vi "Main.vi"(11 "Module Admin":refnum<class "Delacor_lib_QMH_Module Admin.lvclass">) -> ()   [LabVIEW 2026, in "Plaintext to CW Sender.lvlib"]
doc: "This template is based off of the Queued Message Handler design pattern and the Queued Message Handler project template that ships with LabVIEW.\n\nThe main difference is that the queue is private to this module and communication between modules is performed via Broadcast and Request events.\n\nRequest events are wrapped in public API methods and are handled in the Event Handling Loop (EHL) of this VI. Any module can register for Broadcast events sent by this module. The EHL generates messages based on user interface actions.\n\nThe Message Handling Loop (MHL) processes messages generated by the EHL, or by other messages. The messages are string values, so new messages can be added easily to the Message Cases case structure in the MHL. Each message cluster can also provide an optional value for Message Data, which is a variant that can be converted to whatever message-specific data is required.\n_____\nBased on DQMH Dev Tools: Project Template 7.1.2.1547."
uses:
  Plaintext to CW Sender.lvlib
  <vilib>/Delacor/Delacor QMH/Libraries/Module Admin_class/Delacor_lib_QMH_Module Admin.lvclass
  Module Data--cluster.ctl
  <vilib>/Dataflow_G/G-Audio/Controls/Audio Device Refnum.ctl
  <vilib>/Delacor/Delacor QMH/Libraries/Message Queue_class/Delacor_lib_QMH_Message Queue.lvclass/Delacor_lib_QMH_Message Queue.ctl
  Stop Argument--cluster.ctl
  <vilib>/Delacor/Delacor QMH/Libraries/Module Admin_class/Delacor_lib_QMH_Module Admin.lvclass/Delacor_lib_QMH_Module Admin.ctl
  Get VI Ref Argument--cluster.ctl
  Get VI Ref (Reply Payload)--cluster.ctl
  <vilib>/Utility/miscctls.llb/LVPointTypeDef.ctl
  <vilib>/Dataflow_G/G-Audio/Controls/Audio Device Info.ctl
  <vilib>/Dataflow_G/G-Audio/Controls/Audio Device Type.ctl
  <vilib>/Dataflow_G/G-Audio/Controls/Audio Device Native Data Format.ctl
  <vilib>/Dataflow_G/G-Audio/Controls/Audio Device Format.ctl
  <vilib>/Dataflow_G/G-Audio/Controls/Audio Device Config.ctl
  <vilib>/Delacor/Delacor QMH/Libraries/Message Queue_class/Delacor_lib_QMH_Enqueue Message (Single).vi
  <vilib>/Delacor/Delacor QMH/Libraries/Module Admin_class/Delacor_lib_QMH_Get External Launch.vi
  28860a4c-ef95-4274-8184-17b162956eb9.vi
  a59a87ba-3734-490d-884d-561db4356e67.vi
  <vilib>/Dataflow_G/G-Audio/Private/Result To Error.vi
  28860a4c-ef95-4274-8184-17b162956eb9.vi/4dfb5711-8d81-45a3-b3db-a84d40650863.vi
  28860a4c-ef95-4274-8184-17b162956eb9.vi/c8869513-30c6-44f2-a2d3-73232fe63870.vi
  <vilib>/Dataflow_G/G-Audio/Private/Audio Device Refnum To Value.vi
  a59a87ba-3734-490d-884d-561db4356e67.vi/4dfb5711-8d81-45a3-b3db-a84d40650863.vi
  a59a87ba-3734-490d-884d-561db4356e67.vi/c8869513-30c6-44f2-a2d3-73232fe63870.vi
  28860a4c-ef95-4274-8184-17b162956eb9.vi/4dfb5711-8d81-45a3-b3db-a84d40650863.vi/4b7b629c-2e91-4160-9820-a26af8f6e677.vi
  28860a4c-ef95-4274-8184-17b162956eb9.vi/c8869513-30c6-44f2-a2d3-73232fe63870.vi/4b7b629c-2e91-4160-9820-a26af8f6e677.vi
  a59a87ba-3734-490d-884d-561db4356e67.vi/4dfb5711-8d81-45a3-b3db-a84d40650863.vi/4b7b629c-2e91-4160-9820-a26af8f6e677.vi
  a59a87ba-3734-490d-884d-561db4356e67.vi/c8869513-30c6-44f2-a2d3-73232fe63870.vi/4b7b629c-2e91-4160-9820-a26af8f6e677.vi
  <vilib>/Utility/Data Type/Get Numeric Information.vi
  <vilib>/Waveform/WDTOps.llb/WDT Waveform Duration DBL.vi
  <vilib>/Delacor/Delacor QMH/Libraries/Message Queue_class/Delacor_lib_QMH_Message Queue.lvclass
  <vilib>/Dataflow_G/G-Audio/G-Audio.lvlib
  FT-818 CW Key Control/FT-818 CW Key Control.lvlib
panel:
  in  "CAT Rate":u32=38400
  in  "Radio Comm Port":refnum<visa-resource-name>
  in  "Connect to FT-818":bool
  out "CW Waveform":waveform(dbl)(graph)
  in  "Unit Speed (sec)":dbl=0.13 min=0.0 max=0.5 step=0.01
  in  "Word Gap":u8=7
  in  "Character Gap":u8=3
  in  "Send":bool
  in  "Preview":bool
  in  "Plaintext":string
  out "error out":errorcluster
  out "Status":string
  in  "Simulate MHL Error":bool
  in  "Simulate EHL Error":bool
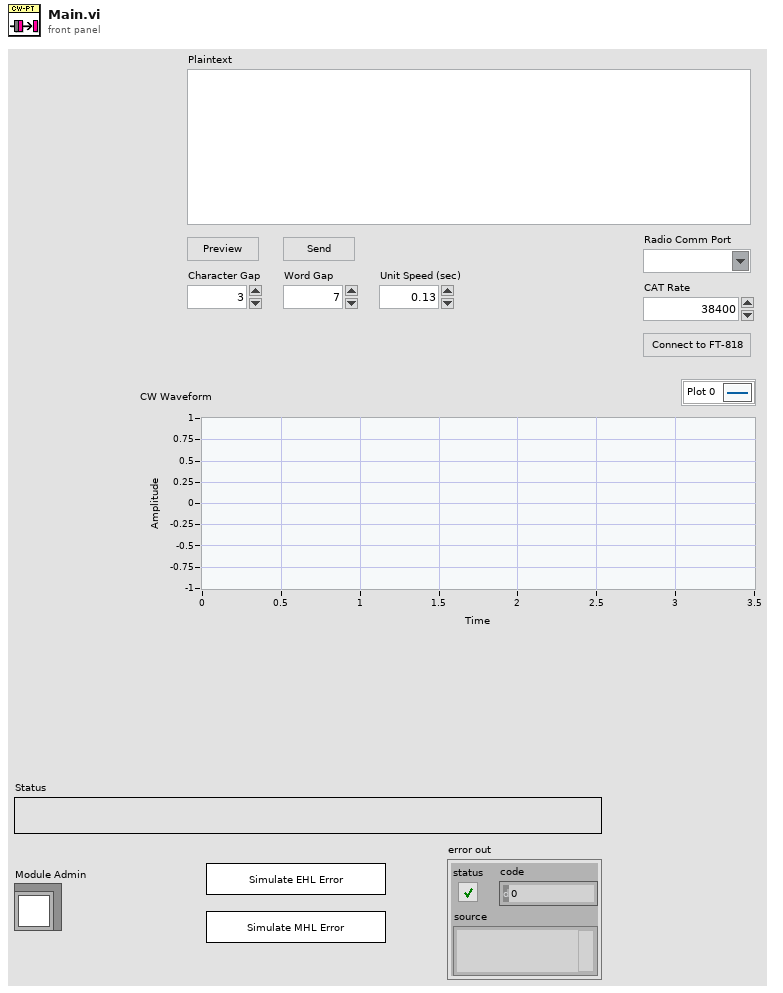
[diagram p1: front panel]
types:
  T1 = typedef "Plaintext to CW Sender.lvlib/Request Events--cluster.ctl" = cluster{"Stop Module":refnum<user-event>, "Show Panel":refnum<user-event>, "Hide Panel":refnum<user-event>, "Get Module Execution Status":refnum<user-event>, "Show Diagram":refnum<user-event>, "Get VI Ref":refnum<user-event>}
  T2 = typedef "FT-818 CW Key Control.lvlib/Broadcast Events--cluster.ctl" = cluster{"Module Did Init":refnum<user-event>, "Status Updated":refnum<user-event>, "Error Reported":refnum<user-event>, "Module Did Stop":refnum<user-event>, "Update Module Execution Status":refnum<user-event>}
  T3 = typedef "Plaintext to CW Sender.lvlib/Module Data--cluster.ctl" = cluster{"Status":string, "Plaintext to CW Map":map{string, bool[]}, "Audio Dev Ref":T4}
  T4 = typedef "G-Audio.lvlib/Audio Device Refnum.ctl" = refnum<file>
  T5 = enum32{"invalid lock state", "Not Locked", "Locked (No Password)", "Password-protected"}
  T6 = typedef "Plaintext to CW Sender.lvlib/Stop Argument--cluster.ctl" = cluster{"Origin":string, "Exit via Stop Module Req?":bool, "Wait for Module to stop?":bool}
  T7 = typedef "Plaintext to CW Sender.lvlib/Get VI Ref Argument--cluster.ctl" = cluster{"Wait Notifier":refnum<notifier>, "wait for reply":bool}
  T8 = typedef "LVPointTypeDef.ctl" = cluster{"Horizontal":i16, "Vertical":i16}
  T9 = enum32{"Invalid", "Standard", "Closed", "Hidden", "Minimized", "Maximized"}
  T10 = typedef "Plaintext to CW Sender.lvlib/Get VI Ref (Reply Payload)--cluster.ctl" = cluster{"VI Refnum":refnum<vi>, "error":errorcluster}
  T11 = typedef "G-Audio.lvlib/Audio Device Config.ctl" = cluster{"Sample Rate (Hz)":u32, "Channels":u32, "Format":T12}
  T12 = typedef "G-Audio.lvlib/Audio Device Format.ctl" = enum16{"Native", "U8", "I16", "I32", "SGL"}
  T13 = typedef "G-Audio.lvlib/Audio Device Info.ctl" = cluster{"Name":string, "ID":u8[], "Device Type":T14, "Default":bool, "Native Data Formats":T15[]}
  T14 = typedef "G-Audio.lvlib/Audio Device Type.ctl" = enum16{"(None)", "Playback", "Capture", "Duplex", "Loopback"}
  T15 = typedef "G-Audio.lvlib/Audio Device Native Data Format.ctl" = cluster{"Format":T12, "Channels":u32, "Sample Rate (Hz)":u32, "Exclusive Mode":bool}
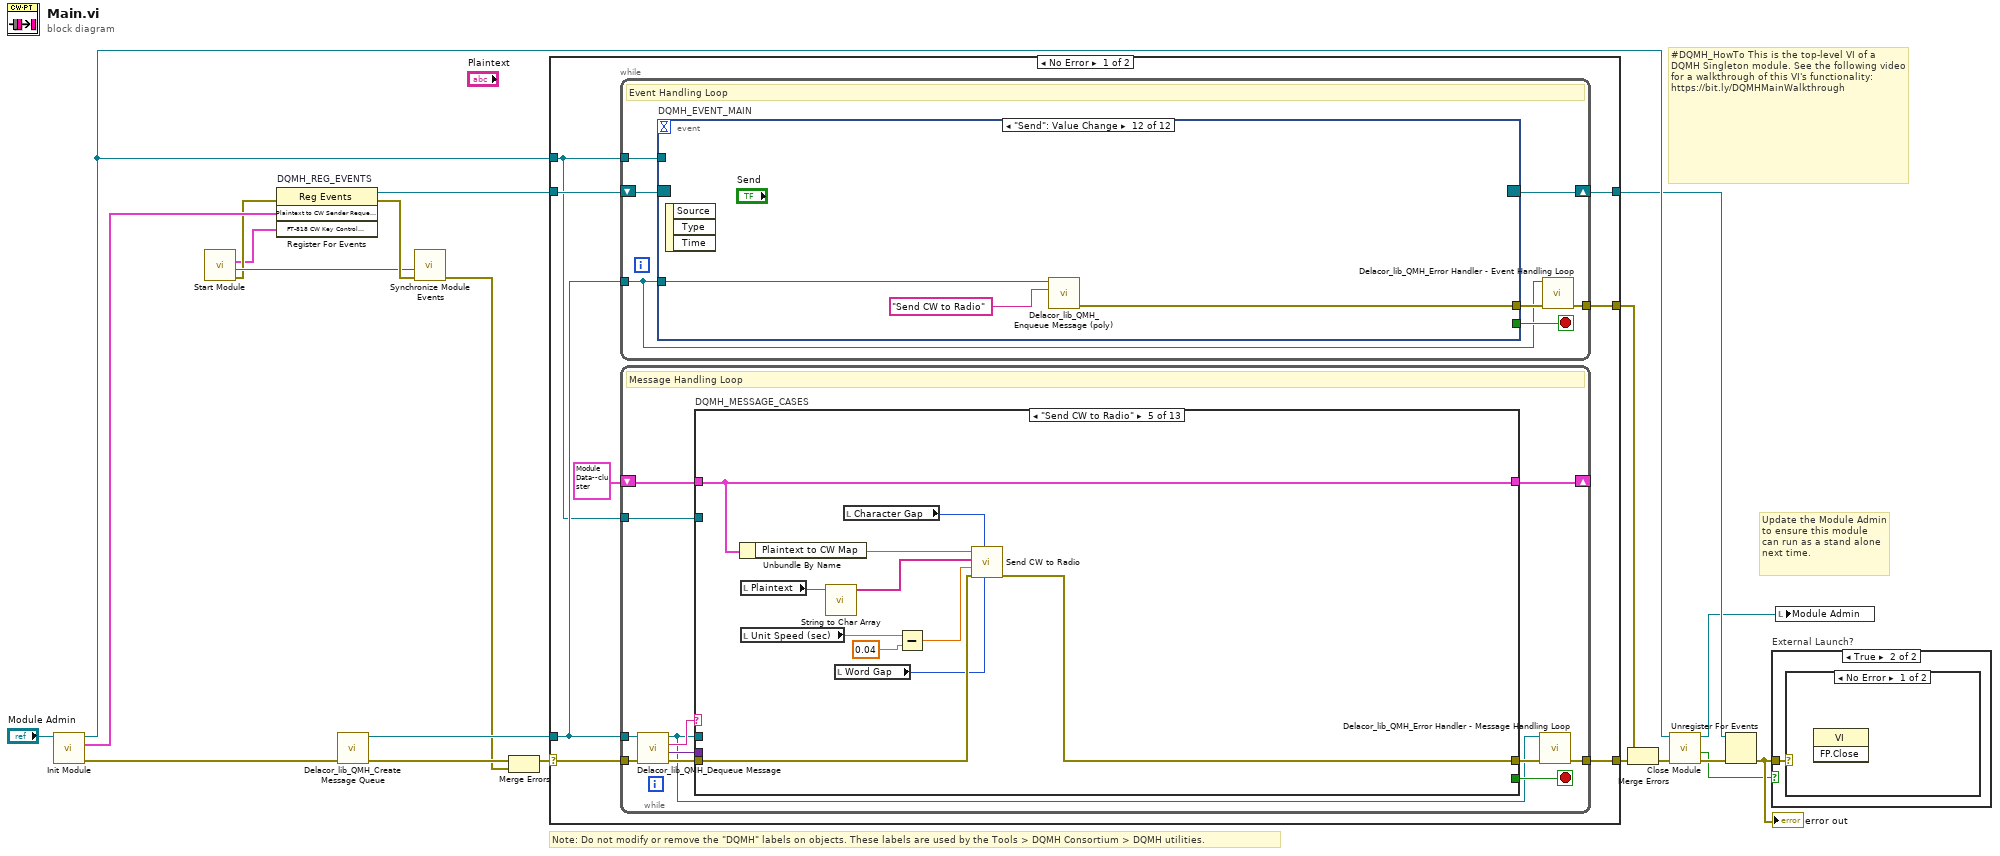
[diagram p0: block diagram]
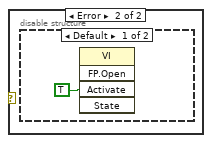
[diagram p3: hidden frame]
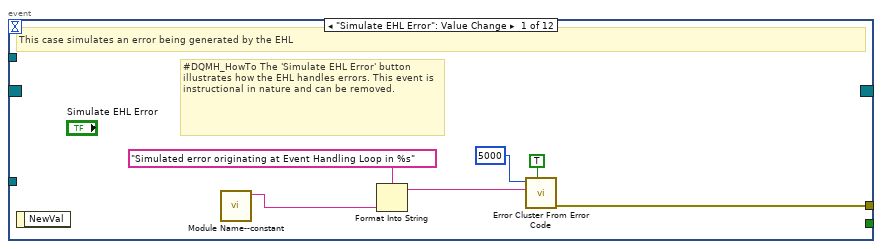
[diagram p5: hidden frame]
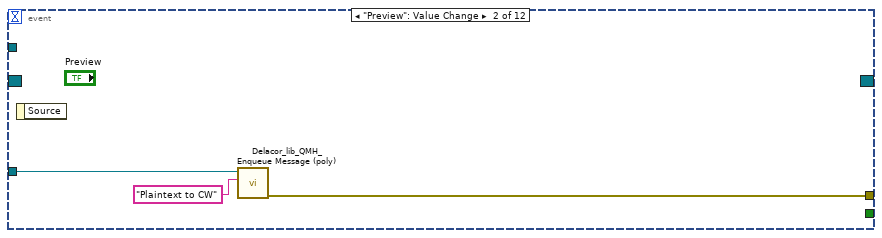
[diagram p6: hidden frame]
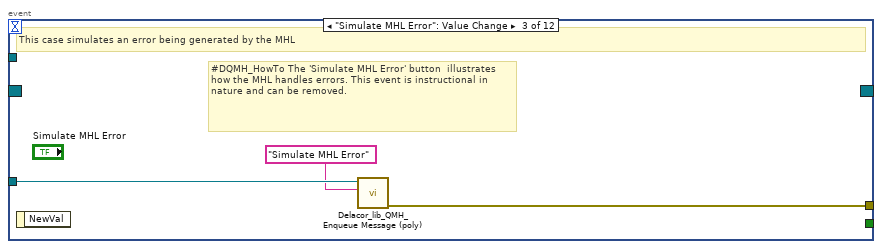
[diagram p7: hidden frame]
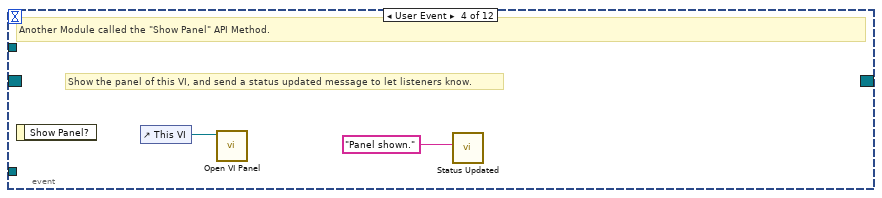
[diagram p8: hidden frame]
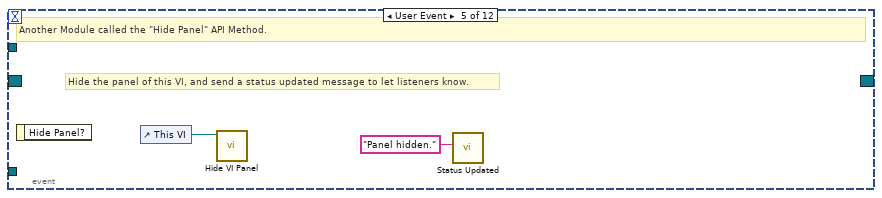
[diagram p9: hidden frame]
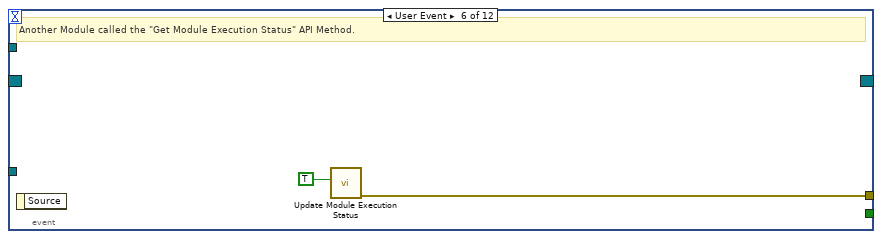
[diagram p10: hidden frame]
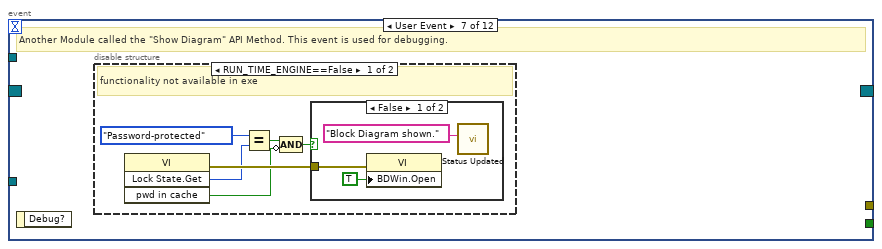
[diagram p11: hidden frame]
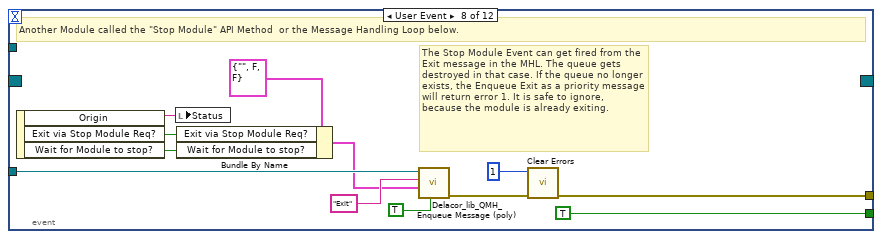
[diagram p14: hidden frame]
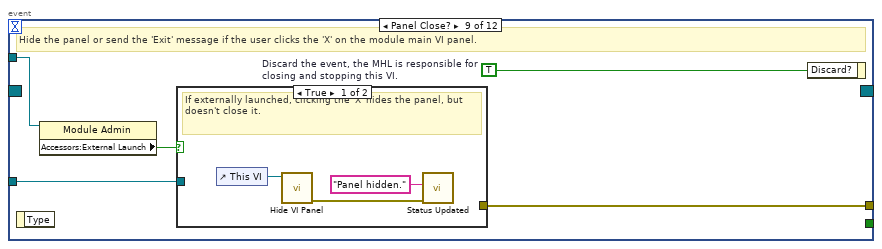
[diagram p15: hidden frame]
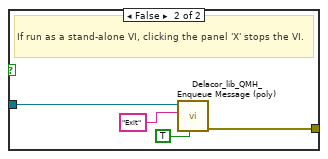
[diagram p16: hidden frame]
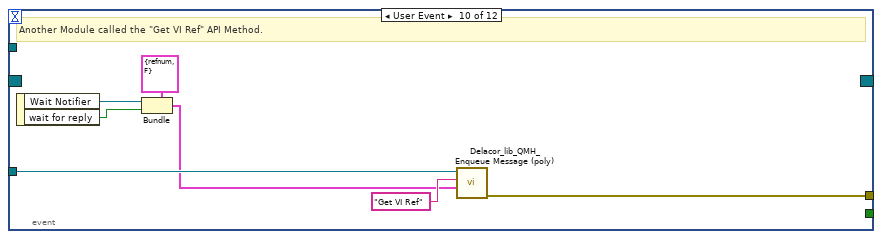
[diagram p17: hidden frame]
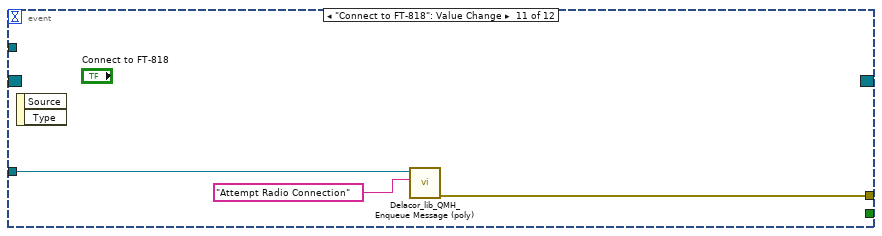
[diagram p18: hidden frame]
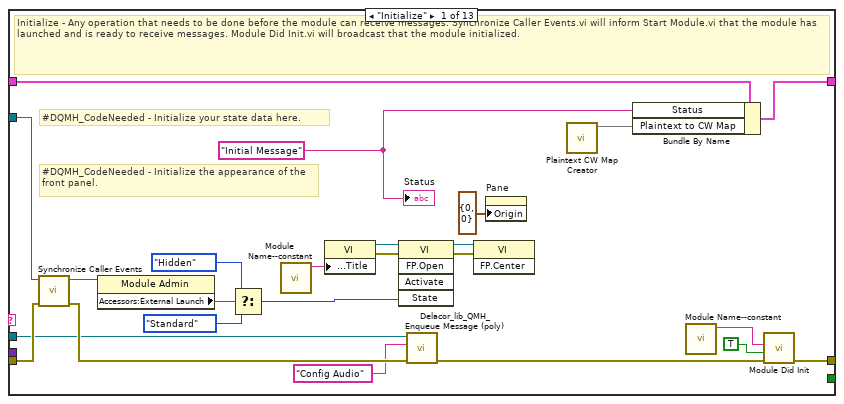
[diagram p19: hidden frame]
diagram:
  # "#DQMH_HowTo This is the top-level VI of a DQMH Singleton module. See the following video for a walkthrough of this VI's functionality: https://bit.ly/DQMHMainWalkthrough"
  # "Note: Do not modify or remove the \"DQMH\" labels on objects. These labels are used by the Tools > DQMH Consortium > DQMH utilities."
  # "Update the Module Admin to ensure this module can run as a stand alone next time."
  n1 = call "Init Module.vi"("Singleton Module Admin in"="Module Admin") -> ("error out"=w20:errorcluster, "Plaintext to CW Sender Request Events"=w10:T1, "Singleton Module Admin out"=w13:refnum<class "Delacor_lib_QMH_Module Admin.lvclass">)  [unwired: 8 in]
  n2 = call "Start Module.vi"() -> ("error out"=w2:errorcluster, "Wait for Event Sync?"=w3:bool, "FT-818 CW Key Control Broadcast Events"=w1:T2)  [unwired: 7 in, 2 out]
  n3 = register-events "DQMH_REG_EVENTS"(error in=w2, w10, w1) -> (reference out=w11:refnum<event-registration>, error out=w5:errorcluster)  [unwired: 1 in]
  n4 = call <vilib>:"Delacor_lib_QMH_Create Message Queue.vi"("error in"=w20) -> ("error out"=w15:errorcluster, "Message Queue"=w9:refnum<class "Delacor_lib_QMH_Message Queue.lvclass">)  [unwired: 9 in]
  n5 = call "Synchronize Module Events.vi"("error in"=w5, "Wait for Event Sync?"=w3) -> ("error out"=w4:errorcluster)  [unwired: 9 in]
  n6 = Merge Errors(w15, w4) -> (w14:errorcluster)
  n7 = case shown="No Error" w14 {
    selector: w14 -> [w27 w269]
    tunnel: [w29 w268] -> w21
    tunnel: [w26 w267] -> w12
    tunnel: w11 -> [w24 w267]
    tunnel: w9 -> [w23 w262]
    tunnel: [w28 _] -> w18
    tunnel: w13 -> [w22 w263]
    frame No Error {
      n8 = while {
        tunnel: w23 -> [w30]
        shift-right: [w33] -> w26
        shift-left: w24 -> [w34]
        tunnel: [w35] -> w28
        tunnel: w22 -> [w31]
        stop <- w32 stop-if-true
        # "Event Handling Loop"
        n9 = event "DQMH_EVENT_MAIN" shown="[11] \"Send\": Value Change" {
          selector: w34 -> [_ _ _ _ _ _ _ _ _ _ _ _]
          dyn-events: [_ _ _ _ _ _ _ _ _ _ _ _] -> w33
          timeout: _ -> [_ _ _ _ _ _ _ _ _ _ _ _]
          tunnel: [_ _ _ _ _ _ _ TRUE ("Discard?") _ _ _ _] -> w32
          tunnel: w30 -> [_ w45 w47 _ _ _ _ w71 w78 w94 w96 w100]
          tunnel: [w42 w44 w48 _ _ w54 _ w74 w80 w88 w97 w99] -> w36
          tunnel: w31 -> [_ _ _ _ _ _ _ _ w77 _ _ _]
          event "Simulate EHL Error": Value Change {
            # "#DQMH_HowTo The 'Simulate EHL Error' button  illustrates how the EHL handles errors. This event is instructional in nature and can be removed."
            # "This case simulates an error being generated by the EHL"
            n10 = event-data() -> ()  [unwired: 1 in, 1 out]
            n11 = call "Module Name--constant.vi"() -> ("Module Name"=w39:string)  [unwired: 11 in]
            n12 = Format Into String(format string="Simulated error originating at Event Handling Loop in %s", w39) -> (resulting string=w40:string)  [unwired: 2 in, 1 out]
            n13 = call <vilib>:"Error Cluster From Error Code.vi"("show call chain? (False)"=TRUE, "error message (\"\")"=w40, "error code (0)"=5000) -> ("error out"=w42:errorcluster)  [unwired: 6 in]
          }
          event "Preview": Value Change {
            n14 = event-data() -> ()  [unwired: 1 in, 1 out]
            n15 = call-poly <vilib>:"Delacor_lib_QMH_Enqueue Message (poly).vi"("Message"="Plaintext to CW", "Message Queue in"=w45) -> ("error out"=w44:errorcluster)  [unwired: 8 in, 1 out]
          }
          event "Simulate MHL Error": Value Change {
            # "#DQMH_HowTo The 'Simulate MHL Error' button  illustrates how the MHL handles errors. This event is instructional in nature and can be removed."
            # "This case simulates an error being generated by the MHL"
            n16 = event-data() -> ()  [unwired: 1 in, 1 out]
            n17 = call-poly <vilib>:"Delacor_lib_QMH_Enqueue Message (poly).vi"("Message"="Simulate MHL Error", "Message Queue in"=w47) -> ("error out"=w48:errorcluster)  [unwired: 8 in, 1 out]
          }
          event User Event {
            # "Show the panel of this VI, and send a status updated message to let listeners know."
            # "Another Module called the \"Show Panel\" API Method."
            n18 = event-data() -> ()  [unwired: 1 in, 1 out]
            n19 = control-ref of="This VI"() -> (w50:refnum<vi>)
            n20 = call "Open VI Panel.vi"("VI"=w50) -> ()  [unwired: 10 in, 1 out]
            n21 = call "Status Updated.vi"("Status"="Panel shown." ("format string")) -> ()  [unwired: 10 in, 1 out]
          }
          event User Event {
            # "Hide the panel of this VI, and send a status updated message to let listeners know."
            # "Another Module called the \"Hide Panel\" API Method."
            n22 = event-data() -> ()  [unwired: 1 in, 1 out]
            n23 = control-ref of="This VI"() -> (w52:refnum<vi>)
            n24 = call "Hide VI Panel.vi"("VI"=w52) -> ()  [unwired: 10 in, 1 out]
            n25 = call "Status Updated.vi"("Status"="Panel hidden." ("format string")) -> ()  [unwired: 10 in, 1 out]
          }
          event User Event {
            # "Another Module called the \"Get Module Execution Status\" API Method."
            n26 = event-data() -> ()  [unwired: 1 in, 1 out]
            n27 = call "Update Module Execution Status.vi"("Running?"=TRUE) -> ("error out"=w54:errorcluster)  [unwired: 10 in]
          }
          event User Event {
            # "Another Module called the \"Show Diagram\" API Method. This event is used for debugging."
            n28 = event-data() -> ()  [unwired: 1 in, 1 out]
            n29 = disable-structure shown="RUN_TIME_ENGINE==False" {
              frame condition #0 (active) {
                # "functionality not available in exe"
                n30 = invoke on="Invoke Node" class="VI" method="Lock State.Get"() -> (error out=w60:errorcluster, "Get Lock State"=w59:T5, "pwd in cache"=w56:bool)  [unwired: 4 in, 1 out]
                n31 = Equal?(x=T5."Password-protected", y=w59) -> (x = y?=w57:bool)
                n32 = Compound Arithmetic op=AND(w57, invert w56) -> (w55:bool)
                n33 = case shown="False" w55 {
                  tunnel: w60 -> [w63 _]
                  frame False {
                    n34 = property on="Property Node" class="VI"(error in=w63, "BDWin.Open"=TRUE ("Block Diagram Window:Open")) -> ()  [unwired: 1 in, 2 out]
                    n35 = call "Status Updated.vi"("Status"="Block Diagram shown." ("format string")) -> ()  [unwired: 10 in, 1 out]
                  }
                  frame True {
                    # "Password-protected VI, and the password is not in the cache. Do not show the diagram."
                  }
                }
              }
              frame condition #1 {
              }
            }
          }
          event User Event {
            # "The Stop Module Event can get fired from the Exit message in the MHL. The queue gets destroyed in that case. If the queue no longer exists, the Enqueue Exit as a priority message will return error 1. It is safe to ignore, because the module is already exiting."
            # "Another Module called the \"Stop Module\" API Method  or the Message Handling Loop below."
            n36 = event-data() -> ("Origin"=w70:string, "Exit via Stop Module Req?"=w66:bool, "Wait for Module to stop?"=w65:bool)  [unwired: 1 in]
            n37 = local write "Status"(w70) -> ()
            n38 = Bundle By Name(cluster=T6 {"Origin"="", "Exit via Stop Module Req?"=FALSE, "Wait for Module to stop?"=FALSE} ("Stop Argument"), "Exit via Stop Module Req?"=w66, "Wait for Module to stop?"=w65) -> (w64:T6)
            n39 = call-poly <vilib>:"Delacor_lib_QMH_Enqueue Message (poly).vi"("Priority Message? (F)"=TRUE, "Message Data"=w64, "Message"="Exit", "Message Queue in"=w71) -> ("error out"=w75:errorcluster)  [unwired: 6 in, 1 out]
            n40 = call <vilib>:"Clear Errors.vi"("error in (no error)"=w75, "specific error code to clear (0: all)"=1) -> ("error out"=w74:errorcluster)  [unwired: 4 in, 1 out]
          }
          event Panel Close? {
            w79 = TRUE  # Discard the event, the MHL is responsible for closing and stopping this VI.
            # "Hide the panel or send the 'Exit' message if the user clicks the 'X' on the module main VI panel."
            n41 = event-data() -> ()  [unwired: 1 in, 1 out]
            n42 = property on="Property Node" class="Module Admin"(reference=w77) -> ("Accessors:External Launch"=w76:bool)  [unwired: 1 in, 2 out]
            n43 = case shown="True" w76 {
              tunnel: w78 -> [_ w86]
              tunnel: [_ w87] -> w80
              frame True {
                # "If externally launched, clicking the 'X' hides the panel, but doesn't close it."
                n44 = control-ref of="This VI"() -> (w83:refnum<vi>)
                n45 = call "Hide VI Panel.vi"("VI"=w83) -> ("error out"=w81:errorcluster)  [unwired: 10 in]
                n46 = call "Status Updated.vi"("error in"=w81, "Status"="Panel hidden." ("format string")) -> ()  [unwired: 9 in, 1 out]
              }
              frame False {
                # "If run as a stand-alone VI, clicking the panel 'X' stops the VI."
                n47 = call-poly <vilib>:"Delacor_lib_QMH_Enqueue Message (poly).vi"("Priority Message? (F)"=TRUE, "Message"="Exit", "Message Queue in"=w86) -> ("error out"=w87:errorcluster)  [unwired: 7 in, 1 out]
              }
            }
            n48 = event-data ("Event Filter Node")("Discard?"=w79) -> ()  [unwired: 1 in, 1 out]
          }
          event User Event {
            # "Another Module called the \"Get VI Ref\" API Method."
            n49 = event-data() -> ("Wait Notifier"=w90:refnum<notifier>, "wait for reply"=w89:bool)  [unwired: 1 in]
            n50 = Bundle(cluster=T7 {"Wait Notifier"=refnum, "wait for reply"=FALSE} ("Get VI Ref Argument"), "Wait Notifier"=w90, "wait for reply"=w89) -> (w91:T7)
            n51 = call-poly <vilib>:"Delacor_lib_QMH_Enqueue Message (poly).vi"("Message Data"=w91, "Message"="Get VI Ref", "Message Queue in"=w94) -> ("error out"=w88:errorcluster)  [unwired: 7 in, 1 out]
          }
          event "Connect to FT-818": Value Change {
            n52 = event-data() -> ()  [unwired: 1 in, 2 out]
            n53 = call-poly <vilib>:"Delacor_lib_QMH_Enqueue Message (poly).vi"("Message"="Attempt Radio Connection", "Message Queue in"=w96) -> ("error out"=w97:errorcluster)  [unwired: 8 in, 1 out]
          }
          event "Send": Value Change {
            n54 = event-data() -> ()  [unwired: 1 in, 3 out]
            n55 = call-poly <vilib>:"Delacor_lib_QMH_Enqueue Message (poly).vi"("Message"="Send CW to Radio", "Message Queue in"=w100) -> ("error out"=w99:errorcluster)  [unwired: 8 in, 1 out]
          }
        }
        n56 = call-dynamic "Delacor_lib_QMH_Error Handler - Event Handling Loop.vi"("error in"=w36, "Message Queue in"=w30) -> ("dup error in"=w35:errorcluster)  [unwired: 8 in, 1 out]
      }
      n57 = while {
        tunnel: w23 -> [w101]
        shift-right: [w109] -> _
        shift-left: T3 {"Status"="", "Plaintext to CW Map"={}, "Audio Dev Ref"=refnum} ("Data Cluster") -> [w110]
        tunnel: w27 -> [w112]
        tunnel: [w104] -> w29
        tunnel: w22 -> [w105]
        stop <- w108 stop-if-true
        # "Message Handling Loop"
        n58 = call-dynamic "Delacor_lib_QMH_Dequeue Message.vi"("error in"=w112, "Message Queue in"=w101) -> ("error out"=w111:errorcluster, "Message Data"=w106:variant, "Message"=w107:string, "Message Queue out"=w102:refnum<class "Delacor_lib_QMH_Message Queue.lvclass">)  [unwired: 6 in]
        n59 = case "DQMH_MESSAGE_CASES" shown="\"Send CW to Radio\"" w107 {
          selector: w107 -> [_ _ _ _ _ _ _ _ _ _ _ _ w257]
          tunnel: w102 -> [w114 _ _ _ _ _ _ _ _ _ w218 w245 _]
          tunnel: w111 -> [w134 w138 w150 w155 w162 w168 w189 w198 w205 w214 w225 w251 w260]
          tunnel: [w132 w138 w141 w154 w161 w167 w175 w193 w205 w213 w221 w246 w261] -> w103
          tunnel: w110 -> [w123 w137 w149 w153 w166 w171 w173 w192 w204 w211 w220 w237 w258]
          tunnel: [w122 w137 w149 w153 w166 w171 w172 w192 w204 w211 w220 w237 w258] -> w109
          tunnel: [_ _ _ _ _ _ _ _ _ _ _ w244 _] -> w108
          tunnel: w106 -> [_ _ w148 _ _ _ _ _ _ _ w219 w243 _]
          tunnel: w105 -> [w124 _ _ _ _ _ _ _ _ _ w217 w238 _]
          frame "Initialize" {
            w118 = "Initial Message" ("Initial Message")
            # "#DQMH_CodeNeeded - Initialize the appearance of the front panel."
            # "#DQMH_CodeNeeded - Initialize your state data here."
            # "Initialize - Any operation that needs to be done before the module can receive messages. Synchronize Caller Events.vi will inform Start Module.vi that the module has launched and is ready to receive messages. Module Did Init.vi will broadcast that the module initialized."
            n60 = call "Synchronize Caller Events.vi"("error in"=w134, "Singleton Module Admin in"=w124) -> ("error out"=w133:errorcluster, "Singleton Module Admin out"=w119:refnum<class "Delacor_lib_QMH_Module Admin.lvclass">)  [unwired: 8 in]
            n61 = property on="Property Node" class="Module Admin"(reference=w119) -> ("Accessors:External Launch"=w128:bool)  [unwired: 1 in, 2 out]
            n62 = Select(t=T9."Hidden" ("State"), s=w128, f=T9."Standard" ("State")) -> (s? t:f=w125:T9)
            n63 = call "Module Name--constant.vi"() -> ("Module Name"=w131:string)  [unwired: 11 in]
            n64 = property on="Property Node" class="VI"("Front Panel.Title"=w131) -> (reference out=w130:refnum<vi>, error out=w136:errorcluster)  [unwired: 2 in]
            n65 = invoke on="Invoke Node" class="VI" method="FP.Open"(reference=w130, error in=w136, "State"=w125) -> (reference out=w129:refnum<vi>, error out=w135:errorcluster)  [unwired: 2 in, 3 out]
            n66 = call-poly <vilib>:"Delacor_lib_QMH_Enqueue Message (poly).vi"("error in"=w133, "Message"="Config Audio", "Message Queue in"=w114) -> ("error out"=w115:errorcluster)  [unwired: 7 in, 1 out]
            n67 = invoke on="Invoke Node" class="VI" method="FP.Center"(reference=w129, error in=w135) -> ()  [unwired: 1 in, 3 out]
            n68 = property on="Pane" class="Pane"("Origin"=T8 {"Horizontal"=0, "Vertical"=0}) -> ()  [unwired: 2 in, 2 out]
            n69 = call "Plaintext CW Map Creator.vi"() -> ("Plaintext to CW Map"=w116:map{string, bool[]})  [unwired: 11 in]
            n70 = Bundle By Name(cluster=w123, "Status"=w118, "Plaintext to CW Map"=w116) -> (w122:T3)
            n71 = call "Module Name--constant.vi"() -> ("Module Name"=w120:string)  [unwired: 11 in]
            n72 = call "Module Did Init.vi"("error in"=w115, "Initialized?"=TRUE, "Origin"=w120) -> ("error out"=w132:errorcluster)  [unwired: 8 in]
            "Status" <- w118
          }
          frame "---Module Specific---" {
            # "Separator -- The following cases handle messages specific to this Module."
          }
          frame "Get VI Ref" {
            # "Returns the VI ref. Usually used for inserting into subVI."
            n73 = Variant To Data(error in=w150, type=T7 {"Wait Notifier"=refnum, "wait for reply"=FALSE} ("Get VI Ref Argument"), Variant=w148) -> (data=w146:T7, error out=w139:errorcluster)
            n74 = Unbundle By Name(w146) -> ("Wait Notifier"=w145:refnum<notifier>, "wait for reply"=w144:bool)
            n75 = control-ref of="This VI"() -> (w140:refnum<vi>)
            n76 = Bundle By Name(cluster=T10 {"VI Refnum"=refnum, "error"={"status"=FALSE, "code"=0, "source"=""}} ("Get VI Ref (Reply Payload)"), "VI Refnum"=w140, "error"=w139) -> (w143:T10)
            n77 = Merge Errors(w139) -> (w141:errorcluster)
            n78 = case "DQMH_FIRE_NOTIFIER" shown="True" w144 {
              tunnel: w145 -> [_ w152]
              tunnel: w143 -> [_ w151]
              frame False {
              }
              frame True {
                n79 = Send Notification(notification=w151, notifier=w152) -> ()  [unwired: 1 in, 2 out]
              }
            }
          }
          frame "---Copy This Frame---" {
            # "Duplicate this frame when creating new messages.  Change this comment in the duplicated frame to describe this message."
            n80 = Merge Errors(w155) -> (w154:errorcluster)
          }
          frame "Send CW to Radio" {
            n81 = Unbundle By Name(w166) -> ("Plaintext to CW Map"=w165:map{string, bool[]})
            n82 = local read "Plaintext"() -> (w164:string)
            n83 = local read "Unit Speed (sec)"() -> (w160:dbl)
            n84 = call "String to Char Array.vi"("string"=w164) -> ("array of chars"=w163:string[])  [unwired: 10 in]
            n85 = local read "Word Gap"() -> (w158:u8)
            n86 = local read "Character Gap"() -> (w159:u8)
            n87 = Subtract(x=w160, y=0.04) -> (x-y=w157:dbl)
            n88 = call "Send CW to Radio.vi"("Word Gap"=w158, "Character Gap"=w159, "error in"=w162, "Unit Speed (sec)"=w157, "Plaintext Array"=w163, "Plaintext to CW Map"=w165) -> ("error out"=w161:errorcluster)  [unwired: 5 in]
          }
          frame "Attempt Radio Connection" {
            n89 = call "Connect to radio.vi"("error in"=w168, "CAT Rate"="CAT Rate", "Radio Comm Port"="Radio Comm Port") -> ("error out"=w167:errorcluster)  [unwired: 6 in, 2 out]
          }
          frame "Config Audio" {
            # "Write nothing first, to\nprep the buffer? It helps\nfor some reason on the\nfirst execution."
            n90 = call <vilib>:"Configure Audio Device.vi"("Buffer Size (4096)"=60000, "error in (no error)"=w189, "Device Config"=T11 {"Sample Rate (Hz)"=1500, "Channels"=1, "Format"=enum."Native"}, "Audio Device"=T13 {"Name"="", "ID"=[0], "Device Type"=enum."Playback", "Default"=FALSE, "Native Data Formats"=[{"Format"=enum."Native", "Channels"=0, "Sample Rate (Hz)"=1500, "Exclusive Mode"=FALSE}]}) -> ("error out"=w184:errorcluster, "Audio Device Refnum"=w185:T4)  [unwired: 4 in, 2 out]
            n91 = call <vilib>:"Start Audio Device.vi"("error in (no error)"=w184, "Audio Device Refnum In"=w185) -> ("error out"=w183:errorcluster, "Audio Device Refnum Out"=w179:T4)  [unwired: 8 in]
            n92 = call "WF Gap Creator.vi"("error in"=w183, "Character Gap"=u8 1, "Unit Speed"=1000.0) -> ("error out"=w180:errorcluster, "waveform out"=w178:waveform(dbl))  [unwired: 7 in]
            n93 = call "Playback Audio.vim"("error in (no error)"=w180, "Audio Data"=w178, "Audio Device Refnum In"=w179) -> ("error out"=w177:errorcluster, "Audio Device Refnum Out"=w176:T4)  [unwired: 7 in]
            n94 = call <vilib>:"Playback Wait.vi"("error in (no error)"=w177, "Audio Device Refnum In"=w176) -> ("error out"=w175:errorcluster, "Audio Device Refnum Out"=w174:T4)  [unwired: 8 in]
            n95 = Bundle By Name(cluster=w173, "Audio Dev Ref"=w174) -> (w172:T3)
          }
          frame "Plaintext to CW" {
            # "Convert Plaintext to array of T & F values."
            n96 = local read "Plaintext"() -> (w203:string)
            n97 = Unbundle By Name(w192) -> ("Plaintext to CW Map"=w190:map{string, bool[]})
            n98 = call "String to Char Array.vi"("string"=w203) -> ("array of chars"=w202:string[])  [unwired: 10 in]
            n99 = call "CW Waveform Generator.vi"("Word Gap"="Word Gap", "Character Gap"="Character Gap", "error in"=w198, "Unit Speed (sec)"="Unit Speed (sec)", "Plaintext Array"=w202, "Plaintext to CW Map"=w190) -> ("error out"=w196:errorcluster, "CW Waveform"=w197:waveform(dbl))  [unwired: 4 in]
            "CW Waveform" <- w197
            n100 = call-poly <vilib>:"Waveform Duration.vi"("error in (no error)"=w196, "waveform in"=w197) -> ("error out"=w194:errorcluster, "waveform out"=w195:waveform(dbl))  [unwired: 7 in, 1 out]
            n101 = Unbundle By Name(w192) -> ("Audio Dev Ref"=w191:T4)
            n102 = call "Playback Audio.vim"("error in (no error)"=w194, "Audio Data"=w195, "Audio Device Refnum In"=w191) -> ("error out"=w193:errorcluster)  [unwired: 7 in, 1 out]
          }
          frame "---Exit and Error Handling---" {
            # "Separator - The following cases handle errors and exit messages."
          }
          frame "Simulate MHL Error" {
            # "#DQMH_HowTo The 'Simulate MHL Error' button  illustrates how the MHL handles errors. This event is instructional in nature and can be removed."
            # "Simulate an error occurring at the MHL"
            n103 = call "Module Name--constant.vi"() -> ("Module Name"=w207:string)  [unwired: 11 in]
            n104 = Format Into String(format string="Simulated error originating at Message Handling Loop in %s", w207) -> (resulting string=w208:string)  [unwired: 2 in, 1 out]
            n105 = call <vilib>:"Error Cluster From Error Code.vi"("show call chain? (False)"=TRUE, "error message (\"\")"=w208, "error code (0)"=5001) -> ("error out"=w212:errorcluster)  [unwired: 6 in]
            n106 = Merge Errors(w214, w212) -> (w213:errorcluster)
          }
          frame "Error" {
            # "#DQMH_CodeRecommended - If the module is running in standalone mode (External Launch = FALSE), this code will pop up an error dialog and call the 'Exit' message if an error occurs. Add more fine-grained error management here."
            # "Error - Check the error message data and respond accordingly. This message is sent by the \"Error Handler\" VIs at the end of each loop in this application."
            n107 = property on="Property Node" class="Module Admin"(reference=w217) -> ("Accessors:External Launch"=w216:bool)  [unwired: 1 in, 2 out]
            n108 = Variant To Data(error in=w225, type=errorcluster {"status"=FALSE, "code"=0, "source"=""} ("error constant"), Variant=w219) -> (data=w215:errorcluster, error out=w223:errorcluster)
            n109 = local write "error out"(w215) -> ()
            n110 = call "Error Reported.vi"("Error"=w215) -> ()  [unwired: 10 in, 1 out]
            n111 = case shown="False" w216 {
              tunnel: [w230 _] -> w222
              tunnel: w218 -> [w228 _]
              tunnel: w215 -> [w229 _]
              frame False {
                n112 = disable-structure shown="Default" {
                  disable-tunnel: w229 -> [w231 _]
                  frame condition #0 (active) {
                    # "If the module is running standalone, then pop up an error dialog and call the \"Exit\" message."
                    n113 = call <vilib>:"Simple Error Handler.vi"("error in (no error)"=w231) -> ()  [unwired: 4 in, 5 out]
                  }
                  frame condition #1 {
                    # "To prevent the Simple Error Handler VI from being loaded (e.g. when deploying to a Real-Time target), add the Conditional Disable Symbol \"DQMH_Disable_SEH\" to your project and set it to TRUE."
                  }
                }
                n114 = call-poly <vilib>:"Delacor_lib_QMH_Enqueue Message (poly).vi"("Priority Message? (F)"=TRUE, "Message"="Exit", "Message Queue in"=w228) -> ("error out"=w230:errorcluster)  [unwired: 7 in, 1 out]
              }
              frame True {
                # "If the module was launched externally, calling the Error Reported broadcast VI is the only action performed by the \"Error\" message. The module's caller can then process the error appropriately."
              }
            }
            n115 = Merge Errors(w223, w222) -> (w221:errorcluster)
          }
          frame "Exit" {
            w242 = 91  # 91: not all Exit messages will have an argument
            w244 = TRUE  # Stop the VI
            # "Release the message queue reference"
            # "#DQMH_CodeNeeded - Add any required cleanup code here."
            # "Exit - Exit the application."
            n116 = Variant To Data(error in=w251, type=T6 {"Origin"="", "Exit via Stop Module Req?"=FALSE, "Wait for Module to stop?"=FALSE} ("Stop Argument"), Variant=w243) -> (data=w240:T6, error out=w248:errorcluster)
            n117 = call <vilib>:"Clear Errors.vi"("error in (no error)"=w248, "specific error code to clear (0: all)"=w242) -> ("error out"=w250:errorcluster)  [unwired: 4 in, 1 out]
            n118 = control-ref of="This VI"() -> (w239:refnum<vi>)
            n119 = call-dynamic "Delacor_lib_QMH_Release Message Queue.vi"("error in"=w250, "Message Queue"=w245) -> ("error out"=w249:errorcluster)  [unwired: 9 in]
            n120 = call "Handle Exit.vi"("Stop Argument"=w240, "Admin in"=w238, "VI reference"=w239) -> ("error out"=w247:errorcluster)  [unwired: 7 in, 1 out]
            n121 = Unbundle By Name(w237) -> ("Audio Dev Ref"=w236:T4)
            n122 = call <vilib>:"Stop Audio Device.vi"("Audio Device Refnum In"=w236) -> ("error out"=w234:errorcluster, "Audio Device Refnum Out"=w235:T4)  [unwired: 9 in]
            n123 = call "Stop Module.vi"() -> ("error out"=w232:errorcluster)  [unwired: 11 in]
            n124 = call <vilib>:"Clear Audio Device.vi"("error in (no error)"=w234, "Audio Device Refnum In"=w235) -> ("error out"=w233:errorcluster)  [unwired: 9 in]
            n125 = Merge Errors(w233, w232, w249, w247) -> (w246:errorcluster)
            n126 = call "Error Reported.vi"("Error"=w246) -> ()  [unwired: 10 in, 1 out]
          }
          frame Default {
            # "'Default' case only runs if there is a message that isn't defined in any of the other cases.  Output a programming error."
            n127 = call "Module Name--constant.vi"() -> ("Module Name"=w256:string)  [unwired: 11 in]
            n128 = Format Into String(format string="The invalid message string \"%s\" was received in the Message Handling Loop for module \"%s\".", w257, w256) -> (resulting string=w252:string)  [unwired: 2 in, 1 out]
            n129 = call <vilib>:"Error Cluster From Error Code.vi"("show call chain? (False)"=TRUE, "error message (\"\")"=w252, "error code (0)"=1) -> ("error out"=w259:errorcluster)  [unwired: 6 in]
            n130 = Merge Errors(w260, w259) -> (w261:errorcluster)
          }
        }
        n131 = call-dynamic "Delacor_lib_QMH_Error Handler - Message Handling Loop.vi"("error in"=w103, "Message Queue in"=w102) -> ("dup error in"=w104:errorcluster)  [unwired: 8 in, 1 out]
      }
    }
    frame Error {
      # "Synchronize Caller Events.vi will inform Start Module.vi that the module has launched and will let the code calling Start Module.vi register for broadcasts and would permit the caller receive the broadcast that an error occurred at launch time."
      n132 = call-dynamic "Delacor_lib_QMH_Release Message Queue.vi"("error in"=w269, "Message Queue"=w262) -> ("error out"=w268:errorcluster)  [unwired: 9 in]
      n133 = call "Synchronize Caller Events.vi"("Singleton Module Admin in"=w263) -> ("error out"=w270:errorcluster)  [unwired: 9 in, 1 out]
      n134 = call "Module Name--constant.vi"() -> ("Module Name"=w266:string)  [unwired: 11 in]
      n135 = Format Into String(format string="An error occurred during initialization. %s is no longer running.", w266) -> (resulting string=w264:string)  [unwired: 2 in, 1 out]
      n136 = Merge Errors(w268, w270) -> (w271:errorcluster)
      n137 = call "Error Reported.vi"("Additional Information"=w264, "Error"=w271) -> ()  [unwired: 9 in, 1 out]
    }
  }
  n138 = Merge Errors(w18, w21) -> (w17:errorcluster)
  n139 = call "Close Module.vi"("error in"=w17, "Module Admin in"=w13) -> ("error out"=w19:errorcluster, "External Launch"=w6:bool, "Module Admin out"=w7:refnum<class "Delacor_lib_QMH_Module Admin.lvclass">)  [unwired: 7 in]
  n140 = Unregister For Events(event registration refnum=w12, error in=w19) -> (error out=w16:errorcluster)
  "error out" <- w16
  n141 = case "External Launch?" shown="True" w6 {
    tunnel: w16 -> [_ w272]
    frame False {
    }
    frame True {
      n142 = case shown="No Error" w272 {
        frame No Error {
          n143 = invoke on="Invoke Node" class="VI" method="FP.Close"() -> ()  [unwired: 3 in, 3 out]
        }
        frame Error {
          n144 = disable-structure shown="Default" {
            frame condition #0 (active) {
              n145 = invoke class="VI" method="FP.Open"("Activate"=TRUE ("Activate?")) -> ()  [unwired: 4 in, 5 out]
            }
            frame condition #1 {
              # "Don't show panel on error if running inside a built EXE."
            }
          }
        }
      }
    }
  }
  n146 = local write "Module Admin"(w7) -> ()
